vi "macro_vecBuilder4x1FIll.vi"   [LabVIEW 2019, in "Trajectory_Library.lvlib"]
uses:
  Trajectory_Library.lvlib
  MatBuilder_Create.vi
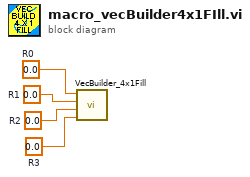
[diagram p0: block diagram]
diagram:
  w1 = 0.0  # R3
  w2 = 0.0  # R2
  w3 = 0.0  # R1
  w4 = 0.0  # R0
  n1 = call "VecBuilder_4x1Fill.vi"("R3"=w1, "R2"=w2, "R1"=w3, "R0"=w4) -> ()  [unwired: 7 in, 1 out]
